vi "FilterDecision.vi"(10 "vHL in":dbl, 11 "vHL 3":sgl) -> (0 "Boolean":bool, 3 "vHL out":dbl)   [LabVIEW 2016]
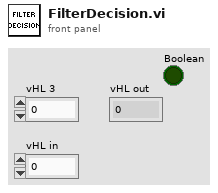
[diagram p1: front panel]
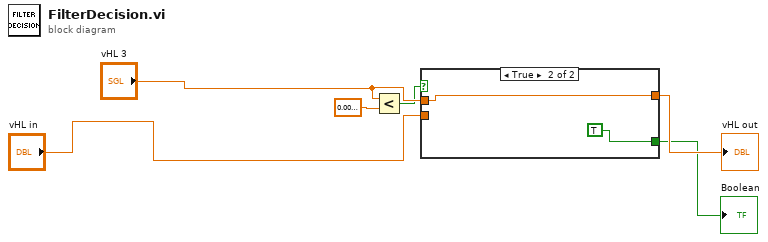
[diagram p0: block diagram]
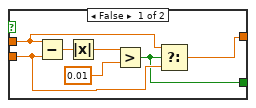
[diagram p2: hidden frame]
diagram:
  n1 = Less?(x="vHL 3", y=sgl 0.01) -> (x < y?=w3:bool)
  n2 = case shown="True" w3 {
    tunnel: "vHL 3" -> [w10 w15]
    tunnel: "vHL in" -> [w9 _]
    tunnel: [w8 w15] -> w6
    tunnel: [w7 TRUE] -> w1
    frame False {
      n3 = Subtract(x=w10, y=w9) -> (x-y=w13:dbl)
      n4 = Absolute Value(x=w13) -> (abs(x)=w11:dbl)
      n5 = Greater?(x=w11, y=0.01) -> (0:w7:bool)
      n6 = Select(t=w10, s=w7, f=w9) -> (s? t:f=w8:dbl)
    }
    frame True {
    }
  }
  "vHL out" <- w6
  "Boolean" <- w1
